vi "核查数据和日志信息出发送队列 (子VI).vi"() -> (0 "错误输出":errorcluster, 3 "核查数据上传":bool)   [LabVIEW 2016, in "数据传输系统.lvlib"]
uses:
  <vilib>/Utility/config.llb/NI_LVConfig.lvlib
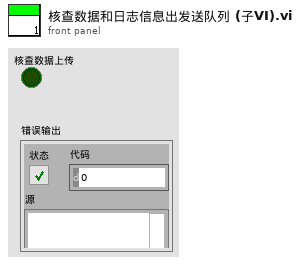
[diagram p1: front panel]
types:
  T1 = enum16{"质控数据", "操作日志", "仪器参数", "系统状态", "运行模式", "测量周期", "超标留样", "报警信息", "环境参数"}
  T2 = enum16{"空白测试", "跨度核查", "标样核查", "加标回收", "平行样", "集成干预"}
  T3 = typedef "NI_LVConfig.lvlib/Config Data RefNum.ctl" = refnum<k1>
  T4 = cluster{"PH":string[][], "CODCr":string[][], "氨氮":string[][], "CODMn":string[][], "总氮":string[][], "总磷":string[][], "电导率":string[][], "水温":string[][], "DO":string[][], "浊度":string[][], "叶绿素":string[][], "藻密度":string[][], "铜":string[][], "盐度":string[][], "水位":string[][], "流速":string[][], "瞬时流量":string[][], "累积流量":string[][]}
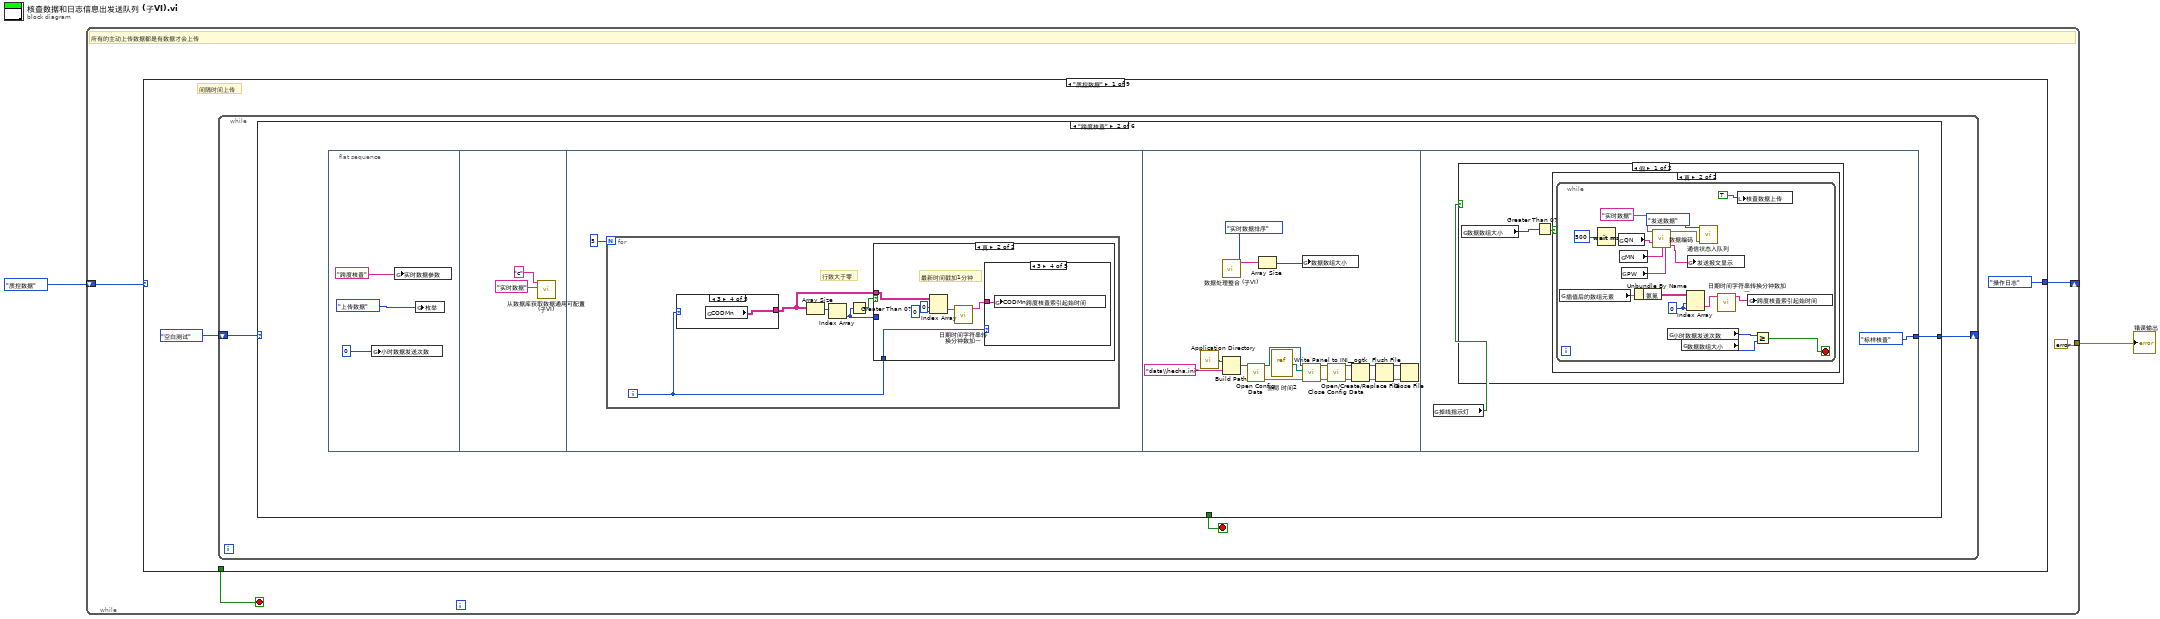
[diagram p0: block diagram]
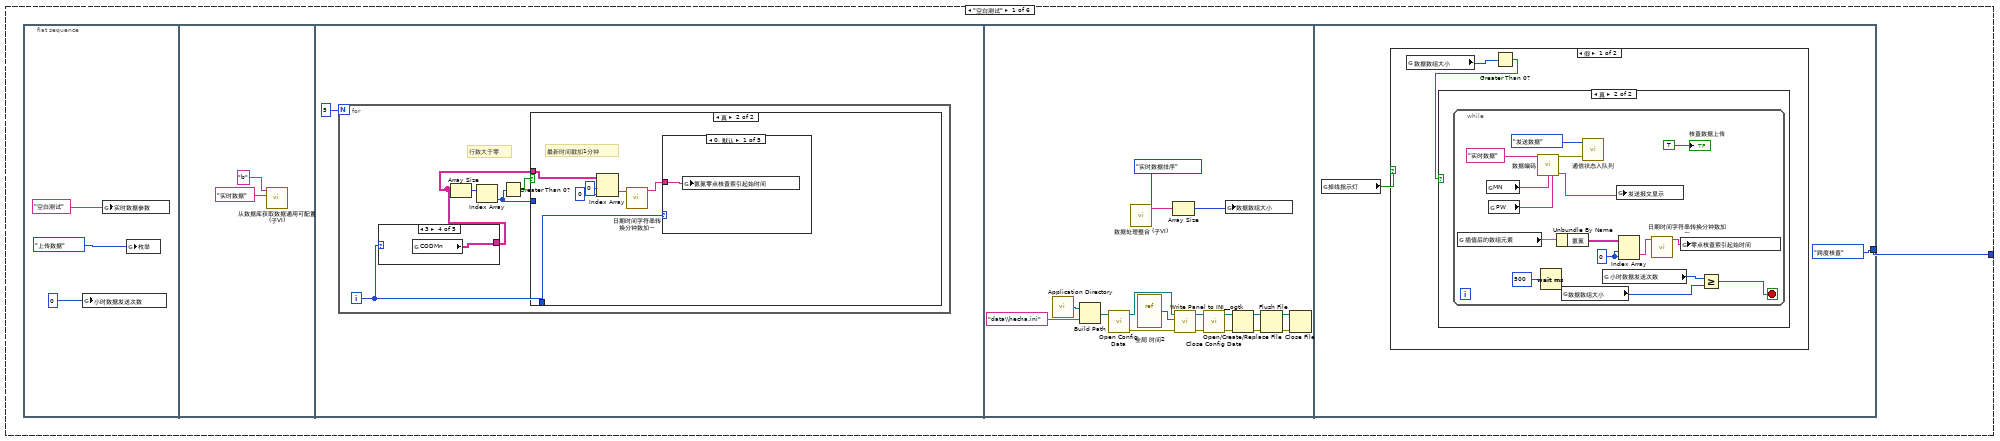
[diagram p2: hidden frame]
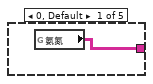
[diagram p3: hidden frame]
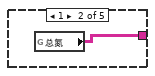
[diagram p4: hidden frame]
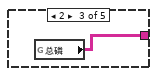
[diagram p5: hidden frame]
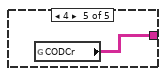
[diagram p6: hidden frame]
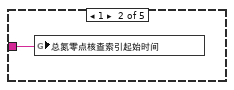
[diagram p8: hidden frame]
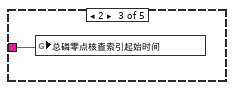
[diagram p9: hidden frame]
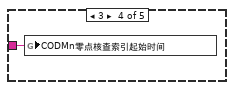
[diagram p10: hidden frame]
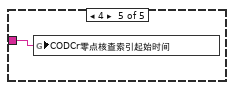
[diagram p11: hidden frame]
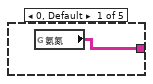
[diagram p14: hidden frame]
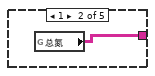
[diagram p15: hidden frame]
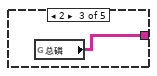
[diagram p16: hidden frame]
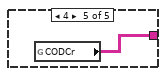
[diagram p17: hidden frame]
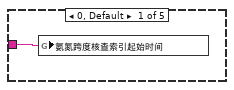
[diagram p19: hidden frame]
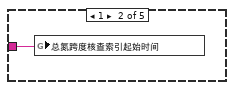
[diagram p20: hidden frame]
diagram:
  n1 = while "While循环" {
    shift-right: [w5] -> _
    shift-left: T1."质控数据" -> [w6]
    tunnel: [errorcluster {"status"=FALSE, "code"=0, "source"=""} ("错误输出")] -> w1
    stop <- w4 stop-if-true
    # "所有的主动上传数据都是有数据才会上传"
    n2 = case shown="\"质控数据\"" w6 {
      tunnel: [T1."操作日志" T1."仪器参数" T1."系统状态" T1."运行模式" T1."测量周期" T1."超标留样" T1."报警信息" T1."环境参数" T1."环境参数"] -> w5
      tunnel: [_ _ _ _ _ _ _ _ TRUE] -> w4
      frame "质控数据" {
        # "间隔时间上传"
        n3 = while {
          shift-right: [w9] -> _
          shift-left: T2."空白测试" -> [w10]
          stop <- w11 stop-if-true
          n4 = case shown="\"跨度核查\"" w10 {
            tunnel: [_ _ _ _ _ TRUE] -> w11
            tunnel: [w12 w77 w143 w173 w205 w266] -> w9
            frame "空白测试" {
              n5 = flat-sequence {
                tunnel: [T2."跨度核查"] -> w12
                frame #0 {
                  n6 = global write "全局 小时数据发送次数.vi" "小时数据发送次数"(0 ("小时数据发送次数")) -> ()
                  n7 = global write "全局 实时数据参数.vi" "实时数据参数"("空白测试") -> ()
                  n8 = global write "全局1.vi" "枚举"(enum16{"返回请求应答", "上传数据", "返回执行结果"}."上传数据" ("枚举")) -> ()
                }
                frame #1 {
                  n9 = call "从数据库获取数据通用可配置(子VI).vi"("table输入"="实时数据" ("新元素/子数组"), "列队名（唯一）"="b") -> ()  [unwired: 8 in, 2 out]
                }
                frame #2 {
                  n10 = for {
                    N: 5 -> [_]
                    i -> [w20]
                    # "行数大于零"
                    n11 = case shown="3" w20 {
                      tunnel: [w24 w25 w26 w27 w28] -> w19
                      frame 0, Default {
                        n12 = global read "全局 所有参数.vi" "氨氮"() -> (w24:string[][])
                      }
                      frame 1 {
                        n13 = global read "全局 所有参数.vi" "总氮"() -> (w25:string[][])
                      }
                      frame 2 {
                        n14 = global read "全局 所有参数.vi" "总磷"() -> (w26:string[][])
                      }
                      frame 3 {
                        n15 = global read "全局 所有参数.vi" "CODMn"() -> (w27:string[][])
                      }
                      frame 4 {
                        n16 = global read "全局 所有参数.vi" "CODCr"() -> (w28:string[][])
                      }
                    }
                    n17 = Array Size(array=w19) -> (size(s)=w22:i32[])
                    n18 = Index Array(array=w22) -> (element=w21:i32)  [unwired: 1 in]
                    n19 = Greater Than 0?(x=w21) -> (x > 0?=w23:bool)
                    n20 = case shown="真" w23 {
                      tunnel: w20 -> [_ w34]
                      tunnel: w21 -> [_ _]
                      tunnel: w19 -> [_ w32]
                      frame False {
                      }
                      frame True {
                        # "最新时间戳加1分钟"
                        n21 = Index Array(array=w32, index (row)=0 ("禁用的索引 (行)"), index (col)=0 ("禁用的索引 (列)")) -> (element=w31:string)
                        n22 = call "日期时间字符串转换分钟数加一.vi"("data[0]"=w31) -> ("日期/时间字符串"=w30:string)  [unwired: 10 in]
                        n23 = case shown="0, 默认" w34 {
                          tunnel: w30 -> [w35 w36 w37 w38 w39]
                          frame 0, Default {
                            n24 = global write "全局 时间2.vi" "氨氮零点核查索引起始时间"(w35) -> ()
                          }
                          frame 1 {
                            n25 = global write "全局 时间2.vi" "总氮零点核查索引起始时间"(w36) -> ()
                          }
                          frame 2 {
                            n26 = global write "全局 时间2.vi" "总磷零点核查索引起始时间"(w37) -> ()
                          }
                          frame 3 {
                            n27 = global write "全局 时间2.vi" "CODMn零点核查索引起始时间"(w38) -> ()
                          }
                          frame 4 {
                            n28 = global write "全局 时间2.vi" "CODCr零点核查索引起始时间"(w39) -> ()
                          }
                        }
                      }
                    }
                  }
                }
                frame #3 {
                  n29 = call <vilib>:"Application Directory.vi"() -> ("Application Directory"=w53:path)
                  n30 = Build Path(base path=w53, name or relative path="data\\hecha.ini" ("名称或相对路径")) -> (appended path=w51:path)
                  n31 = call <vilib>:"Open Config Data.vi"("configuration file path"=w51) -> ("error out"=w47:errorcluster, "refnum"=w50:T3)  [unwired: 8 in, 1 out]
                  n32 = call "数据处理整合 (子VI).vi"("枚举"=enum16{"实时数据排序", "小时数据排序"}."实时数据排序") -> ("已排序的数组"=w56:string[])  [unwired: 10 in]
                  n33 = vi-ref "全局 时间2.vi"() -> (w49:refnum<vi>)
                  n34 = Array Size(array=w56) -> (size(s)=w55:i32)
                  n35 = call <userlib>:"Write Panel to INI__ogtk.vi"("error in (no error)"=w47, "VI ref"=w49, "refnum"=w50) -> ("error out"=w46:errorcluster, "refnum out"=w48:T3)  [unwired: 7 in]
                  n36 = call <vilib>:"Close Config Data.vi"("error in (no error)"=w46, "refnum"=w48) -> ("error out"=w41:errorcluster, "file path"=w40:path)  [unwired: 8 in]
                  n37 = global write "全局 数据数组大小.vi" "数据数组大小"(w55) -> ()
                  n38 = Open/Create/Replace File(file path (use dialog)=w40, error in=w41) -> (refnum out=w44:refnum<file>, error out=w45:errorcluster)  [unwired: 4 in, 1 out]
                  n39 = Flush File(refnum=w44, error in=w45) -> (refnum out=w43:refnum<file>, error out=w42:errorcluster)
                  n40 = Close File(refnum=w43, error in=w42) -> ()  [unwired: 2 out]
                }
                frame #4 {
                  n41 = global read "全局 数据发送重叠.vi" "掉线指示灯"() -> (w58:bool)
                  n42 = case shown="假" w58 {
                    frame False {
                      n43 = global read "全局 数据数组大小.vi" "数据数组大小"() -> (w60:i32)
                      n44 = Greater Than 0?(x=w60) -> (x > 0?=w59:bool)
                      n45 = case shown="真" w59 {
                        frame False {
                        }
                        frame True {
                          n46 = while {
                            stop <- w62 stop-if-true
                            w71 = 0 ("禁用的索引 (列)")
                            n47 = global read "插值后的新数组.vi" "插值后的数组元素"() -> (w75:T4)
                            n48 = global read "断电保存全局.vi" "MN"() -> (w68:string)
                            n49 = global read "断电保存全局.vi" "PW"() -> (w67:string)
                            n50 = call "数据编码.vi"("table输入"="实时数据" ("新元素/子数组"), "MN"=w68, "PW"=w67) -> ("错误常量"=w66:errorcluster, "通讯包字符串"=w70:string)  [unwired: 11 in]
                            n51 = Wait (ms)(milliseconds to wait=u32 500 ("等待时间（毫秒）")) -> ()  [unwired: 1 out]
                            n52 = Unbundle By Name(w75) -> ("氨氮"=w74:string[][])
                            n53 = global read "全局 数据数组大小.vi" "数据数组大小"() -> (w65:i32)
                            n54 = call "通信状态入队列.vi"("错误输入（无错误）"=w66, "枚举"=enum16{"打开连接", "发送数据", "读取数据", "数据处理", "关闭连接"}."发送数据") -> ()  [unwired: 9 in, 1 out]
                            n55 = global read "全局 小时数据发送次数.vi" "小时数据发送次数"() -> (w63:i32)
                            n56 = global write "全局1.vi" "发送报文显示"(w70) -> ()
                            n57 = Index Array(array=w74, index (row)=w71, index (col)=w71) -> (element=w73:string)
                            n58 = call "日期时间字符串转换分钟数加一.vi"("data[0]"=w73) -> ("日期/时间字符串"=w72:string)  [unwired: 10 in]
                            n59 = global write "全局 时间2.vi" "零点核查索引起始时间"(w72) -> ()
                            n60 = Greater Or Equal?(x=w63, y=w65) -> (x >= y?=w62:bool)
                            "核查数据上传" <- TRUE ("数据上传")
                          }
                        }
                      }
                    }
                    frame True {
                    }
                  }
                }
              }
            }
            frame "跨度核查" {
              n61 = flat-sequence {
                tunnel: [T2."标样核查"] -> w77
                frame #0 {
                  n62 = global write "全局 小时数据发送次数.vi" "小时数据发送次数"(0 ("小时数据发送次数")) -> ()
                  n63 = global write "全局 实时数据参数.vi" "实时数据参数"("跨度核查") -> ()
                  n64 = global write "全局1.vi" "枚举"(enum16{"返回请求应答", "上传数据", "返回执行结果"}."上传数据" ("枚举")) -> ()
                }
                frame #1 {
                  n65 = call "从数据库获取数据通用可配置(子VI).vi"("table输入"="实时数据" ("新元素/子数组"), "列队名（唯一）"="c") -> ()  [unwired: 8 in, 2 out]
                }
                frame #2 {
                  n66 = for {
                    N: 5 -> [_]
                    i -> [w84]
                    # "行数大于零"
                    n67 = case shown="3" w84 {
                      tunnel: [w89 w90 w91 w92 w93] -> w85
                      frame 0, Default {
                        n68 = global read "全局 所有参数.vi" "氨氮"() -> (w89:string[][])
                      }
                      frame 1 {
                        n69 = global read "全局 所有参数.vi" "总氮"() -> (w90:string[][])
                      }
                      frame 2 {
                        n70 = global read "全局 所有参数.vi" "总磷"() -> (w91:string[][])
                      }
                      frame 3 {
                        n71 = global read "全局 所有参数.vi" "CODMn"() -> (w92:string[][])
                      }
                      frame 4 {
                        n72 = global read "全局 所有参数.vi" "CODCr"() -> (w93:string[][])
                      }
                    }
                    n73 = Array Size(array=w85) -> (size(s)=w87:i32[])
                    n74 = Index Array(array=w87) -> (element=w86:i32)  [unwired: 1 in]
                    n75 = Greater Than 0?(x=w86) -> (x > 0?=w88:bool)
                    n76 = case shown="真" w88 {
                      tunnel: w84 -> [_ w99]
                      tunnel: w86 -> [_ _]
                      tunnel: w85 -> [_ w97]
                      frame False {
                      }
                      frame True {
                        # "最新时间戳加1分钟"
                        n77 = Index Array(array=w97, index (row)=0 ("禁用的索引 (行)"), index (col)=0 ("禁用的索引 (列)")) -> (element=w96:string)
                        n78 = call "日期时间字符串转换分钟数加一.vi"("data[0]"=w96) -> ("日期/时间字符串"=w95:string)  [unwired: 10 in]
                        n79 = case shown="3" w99 {
                          tunnel: w95 -> [w100 w101 w102 w103 w104]
                          frame 0, Default {
                            n80 = global write "全局 时间2.vi" "氨氮跨度核查索引起始时间"(w100) -> ()
                          }
                          frame 1 {
                            n81 = global write "全局 时间2.vi" "总氮跨度核查索引起始时间"(w101) -> ()
                          }
                          frame 2 {
                            n82 = global write "全局 时间2.vi" "总磷跨度核查索引起始时间"(w102) -> ()
                          }
                          frame 3 {
                            n83 = global write "全局 时间2.vi" "CODMn跨度核查索引起始时间"(w103) -> ()
                          }
                          frame 4 {
                            n84 = global write "全局 时间2.vi" "CODCr跨度核查索引起始时间"(w104) -> ()
                          }
                        }
                      }
                    }
                  }
                }
                frame #3 {
                  n85 = call <vilib>:"Application Directory.vi"() -> ("Application Directory"=w118:path)
                  n86 = call "数据处理整合 (子VI).vi"("枚举"=enum16{"实时数据排序", "小时数据排序"}."实时数据排序") -> ("已排序的数组"=w121:string[])  [unwired: 10 in]
                  n87 = Build Path(base path=w118, name or relative path="data\\hecha.ini" ("名称或相对路径")) -> (appended path=w116:path)
                  n88 = call <vilib>:"Open Config Data.vi"("configuration file path"=w116) -> ("error out"=w112:errorcluster, "refnum"=w115:T3)  [unwired: 8 in, 1 out]
                  n89 = Array Size(array=w121) -> (size(s)=w120:i32)
                  n90 = vi-ref "全局 时间2.vi"() -> (w114:refnum<vi>)
                  n91 = global write "全局 数据数组大小.vi" "数据数组大小"(w120) -> ()
                  n92 = call <userlib>:"Write Panel to INI__ogtk.vi"("error in (no error)"=w112, "VI ref"=w114, "refnum"=w115) -> ("error out"=w111:errorcluster, "refnum out"=w113:T3)  [unwired: 7 in]
                  n93 = call <vilib>:"Close Config Data.vi"("error in (no error)"=w111, "refnum"=w113) -> ("error out"=w106:errorcluster, "file path"=w105:path)  [unwired: 8 in]
                  n94 = Open/Create/Replace File(file path (use dialog)=w105, error in=w106) -> (refnum out=w109:refnum<file>, error out=w110:errorcluster)  [unwired: 4 in, 1 out]
                  n95 = Flush File(refnum=w109, error in=w110) -> (refnum out=w108:refnum<file>, error out=w107:errorcluster)
                  n96 = Close File(refnum=w108, error in=w107) -> ()  [unwired: 2 out]
                }
                frame #4 {
                  n97 = global read "全局 数据发送重叠.vi" "掉线指示灯"() -> (w123:bool)
                  n98 = case shown="假" w123 {
                    frame False {
                      n99 = global read "全局 数据数组大小.vi" "数据数组大小"() -> (w125:i32)
                      n100 = Greater Than 0?(x=w125) -> (x > 0?=w124:bool)
                      n101 = case shown="真" w124 {
                        frame False {
                        }
                        frame True {
                          n102 = while {
                            stop <- w126 stop-if-true
                            w137 = 0 ("禁用的索引 (列)")
                            n103 = global read "插值后的新数组.vi" "插值后的数组元素"() -> (w141:T4)
                            n104 = Wait (ms)(milliseconds to wait=u32 500 ("等待时间（毫秒）")) -> ()  [unwired: 1 out]
                            n105 = global read "全局1.vi" "QN"() -> (w136:string)
                            n106 = global read "断电保存全局.vi" "MN"() -> (w133:string)
                            n107 = global read "断电保存全局.vi" "PW"() -> (w132:string)
                            n108 = Unbundle By Name(w141) -> ("氨氮"=w140:string[][])
                            n109 = call "数据编码.vi"("table输入"="实时数据" ("新元素/子数组"), "QN"=w136, "MN"=w133, "PW"=w132) -> ("错误常量"=w130:errorcluster, "通讯包字符串"=w131:string)  [unwired: 10 in]
                            n110 = global read "全局 小时数据发送次数.vi" "小时数据发送次数"() -> (w127:i32)
                            n111 = global read "全局 数据数组大小.vi" "数据数组大小"() -> (w128:i32)
                            n112 = Index Array(array=w140, index (row)=w137, index (col)=w137) -> (element=w139:string)
                            n113 = global write "全局1.vi" "发送报文显示"(w131) -> ()
                            n114 = call "通信状态入队列.vi"("错误输入（无错误）"=w130, "枚举"=enum16{"打开连接", "发送数据", "读取数据", "数据处理", "关闭连接"}."发送数据") -> ()  [unwired: 9 in, 1 out]
                            n115 = call "日期时间字符串转换分钟数加一.vi"("data[0]"=w139) -> ("日期/时间字符串"=w138:string)  [unwired: 10 in]
                            n116 = local write "核查数据上传"(TRUE ("数据上传")) -> ()
                            n117 = global write "全局 时间2.vi" "跨度核查索引起始时间"(w138) -> ()
                            n118 = Greater Or Equal?(x=w127, y=w128) -> (x >= y?=w126:bool)
                          }
                        }
                      }
                    }
                    frame True {
                    }
                  }
                }
              }
            }
            frame "标样核查" {
              n119 = flat-sequence {
                tunnel: [T2."加标回收"] -> w143
                frame #0 {
                  n120 = global write "全局 小时数据发送次数.vi" "小时数据发送次数"(0 ("小时数据发送次数")) -> ()
                  n121 = global write "全局 实时数据参数.vi" "实时数据参数"("核查数据") -> ()
                  n122 = global write "全局1.vi" "枚举"(enum16{"返回请求应答", "上传数据", "返回执行结果"}."上传数据" ("枚举")) -> ()
                }
                frame #1 {
                  n123 = call "从数据库获取数据通用可配置(子VI).vi"("table输入"="实时数据" ("新元素/子数组"), "列队名（唯一）"="n") -> ()  [unwired: 8 in, 2 out]
                }
                frame #2 {
                  n124 = call "数据处理整合 (子VI).vi"("枚举"=enum16{"实时数据排序", "小时数据排序"}."实时数据排序") -> ("已排序的数组"=w151:string[])  [unwired: 10 in]
                  n125 = Array Size(array=w151) -> (size(s)=w150:i32)
                  n126 = global write "全局 数据数组大小.vi" "数据数组大小"(w150) -> ()
                }
                frame #3 {
                  n127 = global read "全局 数据发送重叠.vi" "掉线指示灯"() -> (w153:bool)
                  n128 = case shown="假" w153 {
                    frame False {
                      n129 = global read "全局 数据数组大小.vi" "数据数组大小"() -> (w155:i32)
                      n130 = Greater Than 0?(x=w155) -> (x > 0?=w154:bool)
                      n131 = case shown="真" w154 {
                        frame False {
                        }
                        frame True {
                          n132 = while {
                            stop <- w157 stop-if-true
                            w167 = 0 ("禁用的索引 (列)")
                            n133 = global read "插值后的新数组.vi" "插值后的数组元素"() -> (w171:T4)
                            n134 = global read "全局1.vi" "QN"() -> (w166:string)
                            n135 = global read "断电保存全局.vi" "MN"() -> (w162:string)
                            n136 = global read "断电保存全局.vi" "PW"() -> (w161:string)
                            n137 = Unbundle By Name(w171) -> ("氨氮"=w170:string[][])
                            n138 = call "数据编码.vi"("table输入"="实时数据" ("新元素/子数组"), "QN"=w166, "MN"=w162, "PW"=w161) -> ("错误常量"=w160:errorcluster, "通讯包字符串"=w165:string)  [unwired: 10 in]
                            n139 = global read "全局 小时数据发送次数.vi" "小时数据发送次数"() -> (w158:i32)
                            n140 = global write "全局1.vi" "发送报文显示"(w165) -> ()
                            n141 = global read "全局 数据数组大小.vi" "数据数组大小"() -> (w159:i32)
                            n142 = Index Array(array=w170, index (row)=w167, index (col)=w167) -> (element=w169:string)
                            n143 = call "通信状态入队列.vi"("错误输入（无错误）"=w160, "枚举"=enum16{"打开连接", "发送数据", "读取数据", "数据处理", "关闭连接"}."发送数据") -> ()  [unwired: 9 in, 1 out]
                            n144 = call "日期时间字符串转换分钟数加一.vi"("data[0]"=w169) -> ("日期/时间字符串"=w168:string)  [unwired: 10 in]
                            n145 = local write "核查数据上传"(TRUE ("数据上传")) -> ()
                            n146 = global write "全局 时间2.vi" "标样核查索引起始时间"(w168) -> ()
                            n147 = Greater Or Equal?(x=w158, y=w159) -> (x >= y?=w157:bool)
                            n148 = Wait (ms)(milliseconds to wait=u32 500 ("等待时间（毫秒）")) -> ()  [unwired: 1 out]
                          }
                        }
                      }
                    }
                    frame True {
                    }
                  }
                }
              }
            }
            frame "加标回收" {
              n149 = flat-sequence {
                tunnel: [T2."平行样"] -> w173
                frame #0 {
                  n150 = global write "全局 小时数据发送次数.vi" "小时数据发送次数"(0 ("小时数据发送次数")) -> ()
                  n151 = global write "全局 实时数据参数.vi" "实时数据参数"("加标回收测试") -> ()
                  n152 = global write "全局1.vi" "枚举"(enum16{"返回请求应答", "上传数据", "返回执行结果"}."上传数据" ("枚举")) -> ()
                }
                frame #1 {
                  n153 = call "从数据库获取数据通用可配置(子VI).vi"("table输入"="加标回收" ("新元素/子数组"), "列队名（唯一）"="d") -> ()  [unwired: 8 in, 2 out]
                }
                frame #2 {
                  n154 = call "加标回收数据处理整合 (子VI).vi"("枚举"=enum16{"实时数据排序", "小时数据排序"}."实时数据排序") -> ("已排序的数组"=w180:string[])  [unwired: 10 in]
                  n155 = Array Size(array=w180) -> (size(s)=w181:i32)
                  n156 = global write "全局 数据数组大小.vi" "数据数组大小"(w181) -> ()
                }
                frame #3 {
                  n157 = global read "全局 数据发送重叠.vi" "掉线指示灯"() -> (w183:bool)
                  n158 = case shown="假" w183 {
                    frame False {
                      n159 = global read "全局 数据数组大小.vi" "数据数组大小"() -> (w185:i32)
                      n160 = Greater Than 0?(x=w185) -> (x > 0?=w184:bool)
                      n161 = case shown="真" w184 {
                        frame False {
                        }
                        frame True {
                          n162 = while {
                            stop <- w187 stop-if-true
                            n163 = global read "全局 数据数组大小.vi" "数据数组大小"() -> (w200:i32)
                            n164 = global read "插值后的新数组.vi" "插值后的数组元素"() -> (w203:T4)
                            n165 = global read "全局1.vi" "QN"() -> (w196:string)
                            n166 = global read "断电保存全局.vi" "MN"() -> (w192:string)
                            n167 = global read "断电保存全局.vi" "PW"() -> (w191:string)
                            n168 = Decrement(x=w200) -> (x-1=w199:i32)
                            n169 = call "数据编码.vi"("table输入"="实时数据" ("新元素/子数组"), "QN"=w196, "MN"=w192, "PW"=w191) -> ("错误常量"=w190:errorcluster, "通讯包字符串"=w195:string)  [unwired: 10 in]
                            n170 = Unbundle By Name(w203) -> ("氨氮"=w202:string[][])
                            n171 = global write "全局1.vi" "发送报文显示"(w195) -> ()
                            n172 = call "通信状态入队列.vi"("错误输入（无错误）"=w190, "枚举"=enum16{"打开连接", "发送数据", "读取数据", "数据处理", "关闭连接"}."发送数据") -> ()  [unwired: 9 in, 1 out]
                            n173 = global read "全局 小时数据发送次数.vi" "小时数据发送次数"() -> (w188:i32)
                            n174 = Index Array(array=w202, index (row)=w199, index (col)=0 ("禁用的索引 (列)")) -> (element=w198:string)
                            n175 = global read "全局 数据数组大小.vi" "数据数组大小"() -> (w189:i32)
                            n176 = call "日期时间字符串转换分钟数加一.vi"("data[0]"=w198) -> ("日期/时间字符串"=w197:string)  [unwired: 10 in]
                            n177 = local write "核查数据上传"(TRUE ("数据上传")) -> ()
                            n178 = global write "全局 时间2.vi" "加标回收索引起始时间"(w197) -> ()
                            n179 = Greater Or Equal?(x=w188, y=w189) -> (x >= y?=w187:bool)
                            n180 = Wait (ms)(milliseconds to wait=u32 500 ("等待时间（毫秒）")) -> ()  [unwired: 1 out]
                          }
                        }
                      }
                    }
                    frame True {
                    }
                  }
                }
              }
            }
            frame "平行样" {
              n181 = flat-sequence {
                tunnel: [T2."集成干预"] -> w205
                frame #0 {
                  n182 = global write "全局 小时数据发送次数.vi" "小时数据发送次数"(0 ("小时数据发送次数")) -> ()
                  n183 = global write "全局 实时数据参数.vi" "实时数据参数"("平行样测试") -> ()
                  n184 = global write "全局1.vi" "枚举"(enum16{"返回请求应答", "上传数据", "返回执行结果"}."上传数据" ("枚举")) -> ()
                }
                frame #1 {
                  n185 = call "从数据库获取数据通用可配置(子VI).vi"("table输入"="平行样测试" ("新元素/子数组"), "列队名（唯一）"="e") -> ()  [unwired: 8 in, 2 out]
                }
                frame #2 {
                  n186 = for {
                    N: 5 -> [_]
                    i -> [w212]
                    # "行数大于零"
                    n187 = case shown="3" w212 {
                      tunnel: [w217 w218 w219 w220 w221] -> w213
                      frame 0, Default {
                        n188 = global read "全局 所有参数.vi" "氨氮"() -> (w217:string[][])
                      }
                      frame 1 {
                        n189 = global read "全局 所有参数.vi" "总氮"() -> (w218:string[][])
                      }
                      frame 2 {
                        n190 = global read "全局 所有参数.vi" "总磷"() -> (w219:string[][])
                      }
                      frame 3 {
                        n191 = global read "全局 所有参数.vi" "CODMn"() -> (w220:string[][])
                      }
                      frame 4 {
                        n192 = global read "全局 所有参数.vi" "CODCr"() -> (w221:string[][])
                      }
                    }
                    n193 = Array Size(array=w213) -> (size(s)=w215:i32[])
                    n194 = Index Array(array=w215) -> (element=w214:i32)  [unwired: 1 in]
                    n195 = Greater Than 0?(x=w214) -> (x > 0?=w216:bool)
                    n196 = case shown="真" w216 {
                      tunnel: w212 -> [_ w227]
                      tunnel: w214 -> [_ _]
                      tunnel: w213 -> [_ w225]
                      frame False {
                      }
                      frame True {
                        # "最新时间戳加1分钟"
                        n197 = Index Array(array=w225, index (row)=0 ("禁用的索引 (行)"), index (col)=0 ("禁用的索引 (列)")) -> (element=w224:string)
                        n198 = call "日期时间字符串转换分钟数加一.vi"("data[0]"=w224) -> ("日期/时间字符串"=w223:string)  [unwired: 10 in]
                        n199 = case shown="0, 默认" w227 {
                          tunnel: w223 -> [w228 w229 w230 w231 w232]
                          frame 0, Default {
                            n200 = global write "全局 时间2.vi" "氨氮平行样索引起始时间"(w228) -> ()
                          }
                          frame 1 {
                            n201 = global write "全局 时间2.vi" "总氮平行样索引起始时间"(w229) -> ()
                          }
                          frame 2 {
                            n202 = global write "全局 时间2.vi" "总磷平行样索引起始时间"(w230) -> ()
                          }
                          frame 3 {
                            n203 = global write "全局 时间2.vi" "CODMn平行样索引起始时间"(w231) -> ()
                          }
                          frame 4 {
                            n204 = global write "全局 时间2.vi" "CODCr平行样索引起始时间"(w232) -> ()
                          }
                        }
                      }
                    }
                  }
                }
                frame #3 {
                  n205 = call "数据处理整合 (子VI).vi"("枚举"=enum16{"实时数据排序", "小时数据排序"}."实时数据排序") -> ("已排序的数组"=w249:string[])  [unwired: 10 in]
                  n206 = Array Size(array=w249) -> (size(s)=w248:i32)
                  n207 = call <vilib>:"Application Directory.vi"() -> ("Application Directory"=w246:path)
                  n208 = Build Path(base path=w246, name or relative path="data\\hecha.ini" ("名称或相对路径")) -> (appended path=w244:path)
                  n209 = global write "全局 数据数组大小.vi" "数据数组大小"(w248) -> ()
                  n210 = call <vilib>:"Open Config Data.vi"("configuration file path"=w244) -> ("error out"=w240:errorcluster, "refnum"=w243:T3)  [unwired: 8 in, 1 out]
                  n211 = vi-ref "全局 时间2.vi"() -> (w242:refnum<vi>)
                  n212 = call <userlib>:"Write Panel to INI__ogtk.vi"("error in (no error)"=w240, "VI ref"=w242, "refnum"=w243) -> ("error out"=w239:errorcluster, "refnum out"=w241:T3)  [unwired: 7 in]
                  n213 = call <vilib>:"Close Config Data.vi"("error in (no error)"=w239, "refnum"=w241) -> ("error out"=w234:errorcluster, "file path"=w233:path)  [unwired: 8 in]
                  n214 = Open/Create/Replace File(file path (use dialog)=w233, error in=w234) -> (refnum out=w237:refnum<file>, error out=w238:errorcluster)  [unwired: 4 in, 1 out]
                  n215 = Flush File(refnum=w237, error in=w238) -> (refnum out=w236:refnum<file>, error out=w235:errorcluster)
                  n216 = Close File(refnum=w236, error in=w235) -> ()  [unwired: 2 out]
                }
                frame #4 {
                  n217 = global read "全局 数据发送重叠.vi" "掉线指示灯"() -> (w250:bool)
                  n218 = case shown="假" w250 {
                    frame False {
                      n219 = global read "全局 数据数组大小.vi" "数据数组大小"() -> (w253:i32)
                      n220 = Greater Than 0?(x=w253) -> (x > 0?=w252:bool)
                      n221 = case shown="真" w252 {
                        frame False {
                        }
                        frame True {
                          n222 = while {
                            stop <- w255 stop-if-true
                            n223 = global read "全局1.vi" "QN"() -> (w264:string)
                            n224 = global read "断电保存全局.vi" "MN"() -> (w260:string)
                            n225 = global read "断电保存全局.vi" "PW"() -> (w259:string)
                            n226 = global read "全局 小时数据发送次数.vi" "小时数据发送次数"() -> (w256:i32)
                            n227 = global read "全局 数据数组大小.vi" "数据数组大小"() -> (w257:i32)
                            n228 = call "数据编码.vi"("table输入"="实时数据" ("新元素/子数组"), "QN"=w264, "MN"=w260, "PW"=w259) -> ("错误常量"=w258:errorcluster, "通讯包字符串"=w263:string)  [unwired: 10 in]
                            n229 = local write "核查数据上传"(TRUE ("数据上传")) -> ()
                            n230 = global write "全局1.vi" "发送报文显示"(w263) -> ()
                            n231 = call "通信状态入队列.vi"("错误输入（无错误）"=w258, "枚举"=enum16{"打开连接", "发送数据", "读取数据", "数据处理", "关闭连接"}."发送数据") -> ()  [unwired: 9 in, 1 out]
                            n232 = Greater Or Equal?(x=w256, y=w257) -> (x >= y?=w255:bool)
                            n233 = Wait (ms)(milliseconds to wait=u32 500 ("等待时间（毫秒）")) -> ()  [unwired: 1 out]
                          }
                        }
                      }
                    }
                    frame True {
                    }
                  }
                }
              }
            }
            frame "集成干预" {
              n234 = flat-sequence {
                tunnel: [T2."集成干预"] -> w266
                frame #0 {
                  n235 = global write "全局 小时数据发送次数.vi" "小时数据发送次数"(0 ("小时数据发送次数")) -> ()
                  n236 = global write "全局 实时数据参数.vi" "实时数据参数"("集成干预测试") -> ()
                  n237 = global write "全局1.vi" "枚举"(enum16{"返回请求应答", "上传数据", "返回执行结果"}."上传数据" ("枚举")) -> ()
                }
                frame #1 {
                  n238 = call "从数据库获取数据通用可配置(子VI).vi"("table输入"="集成干预测试" ("新元素/子数组"), "列队名（唯一）"="f") -> ()  [unwired: 8 in, 2 out]
                }
                frame #2 {
                  n239 = for {
                    N: 10 -> [_]
                    i -> [w274]
                    # "行数大于零"
                    n240 = case shown="9" w274 {
                      tunnel: [w279 w280 w281 w282 w283 w284 w285 w286 w287 w288] -> w275
                      frame 0, Default {
                        n241 = global read "全局 所有参数.vi" "氨氮"() -> (w279:string[][])
                      }
                      frame 1 {
                        n242 = global read "全局 所有参数.vi" "总氮"() -> (w280:string[][])
                      }
                      frame 2 {
                        n243 = global read "全局 所有参数.vi" "总磷"() -> (w281:string[][])
                      }
                      frame 3 {
                        n244 = global read "全局 所有参数.vi" "CODMn"() -> (w282:string[][])
                      }
                      frame 4 {
                        n245 = global read "全局 所有参数.vi" "CODCr"() -> (w283:string[][])
                      }
                      frame 5 {
                        n246 = global read "全局 所有参数.vi" "DO"() -> (w284:string[][])
                      }
                      frame 6 {
                        n247 = global read "全局 所有参数.vi" "PH"() -> (w285:string[][])
                      }
                      frame 7 {
                        n248 = global read "全局 所有参数.vi" "电导率"() -> (w286:string[][])
                      }
                      frame 8 {
                        n249 = global read "全局 所有参数.vi" "水温"() -> (w287:string[][])
                      }
                      frame 9 {
                        n250 = global read "全局 所有参数.vi" "浊度"() -> (w288:string[][])
                      }
                    }
                    n251 = Array Size(array=w275) -> (size(s)=w277:i32[])
                    n252 = Index Array(array=w277) -> (element=w276:i32)  [unwired: 1 in]
                    n253 = Greater Than 0?(x=w276) -> (x > 0?=w278:bool)
                    n254 = case shown="真" w278 {
                      tunnel: w274 -> [_ w294]
                      tunnel: w276 -> [_ _]
                      tunnel: w275 -> [_ w292]
                      frame False {
                      }
                      frame True {
                        # "最新时间戳加1分钟"
                        n255 = Index Array(array=w292, index (row)=0 ("禁用的索引 (行)"), index (col)=0 ("禁用的索引 (列)")) -> (element=w291:string)
                        n256 = call "日期时间字符串转换分钟数加一.vi"("data[0]"=w291) -> ("日期/时间字符串"=w290:string)  [unwired: 10 in]
                        n257 = case shown="9" w294 {
                          tunnel: w290 -> [w295 w296 w297 w298 w299 w300 w301 w302 w303 w304]
                          frame 0, Default {
                            n258 = global write "全局 时间2.vi" "氨氮集成干预索引起始时间"(w295) -> ()
                          }
                          frame 1 {
                            n259 = global write "全局 时间2.vi" "总氮集成干预索引起始时间"(w296) -> ()
                          }
                          frame 2 {
                            n260 = global write "全局 时间2.vi" "总磷集成干预索引起始时间"(w297) -> ()
                          }
                          frame 3 {
                            n261 = global write "全局 时间2.vi" "CODMn集成干预索引起始时间"(w298) -> ()
                          }
                          frame 4 {
                            n262 = global write "全局 时间2.vi" "CODCr集成干预索引起始时间"(w299) -> ()
                          }
                          frame 5 {
                            n263 = global write "全局 时间2.vi" "DO集成干预索引起始时间"(w300) -> ()
                          }
                          frame 6 {
                            n264 = global write "全局 时间2.vi" "PH集成干预索引起始时间"(w301) -> ()
                          }
                          frame 7 {
                            n265 = global write "全局 时间2.vi" "比电导率集成干预索引起始时间"(w302) -> ()
                          }
                          frame 8 {
                            n266 = global write "全局 时间2.vi" "水温集成干预索引起始时间"(w303) -> ()
                          }
                          frame 9 {
                            n267 = global write "全局 时间2.vi" "浊度集成干预索引起始时间"(w304) -> ()
                          }
                        }
                      }
                    }
                  }
                }
                frame #3 {
                  n268 = call "数据处理整合 (子VI).vi"("枚举"=enum16{"实时数据排序", "小时数据排序"}."实时数据排序") -> ("已排序的数组"=w321:string[])  [unwired: 10 in]
                  n269 = Array Size(array=w321) -> (size(s)=w320:i32)
                  n270 = call <vilib>:"Application Directory.vi"() -> ("Application Directory"=w318:path)
                  n271 = Build Path(base path=w318, name or relative path="data\\hecha.ini" ("名称或相对路径")) -> (appended path=w316:path)
                  n272 = global write "全局 数据数组大小.vi" "数据数组大小"(w320) -> ()
                  n273 = call <vilib>:"Open Config Data.vi"("configuration file path"=w316) -> ("error out"=w312:errorcluster, "refnum"=w315:T3)  [unwired: 8 in, 1 out]
                  n274 = vi-ref "全局 时间2.vi"() -> (w314:refnum<vi>)
                  n275 = call <userlib>:"Write Panel to INI__ogtk.vi"("error in (no error)"=w312, "VI ref"=w314, "refnum"=w315) -> ("error out"=w311:errorcluster, "refnum out"=w313:T3)  [unwired: 7 in]
                  n276 = call <vilib>:"Close Config Data.vi"("error in (no error)"=w311, "refnum"=w313) -> ("error out"=w306:errorcluster, "file path"=w305:path)  [unwired: 8 in]
                  n277 = Open/Create/Replace File(file path (use dialog)=w305, error in=w306) -> (refnum out=w309:refnum<file>, error out=w310:errorcluster)  [unwired: 4 in, 1 out]
                  n278 = Flush File(refnum=w309, error in=w310) -> (refnum out=w308:refnum<file>, error out=w307:errorcluster)
                  n279 = Close File(refnum=w308, error in=w307) -> ()  [unwired: 2 out]
                }
                frame #4 {
                  n280 = global read "全局 数据发送重叠.vi" "掉线指示灯"() -> (w323:bool)
                  n281 = case shown="假" w323 {
                    frame False {
                      n282 = global read "全局 数据数组大小.vi" "数据数组大小"() -> (w325:i32)
                      n283 = Greater Than 0?(x=w325) -> (x > 0?=w324:bool)
                      n284 = case shown="真" w324 {
                        frame False {
                        }
                        frame True {
                          n285 = while {
                            stop <- w327 stop-if-true
                            n286 = global read "全局1.vi" "QN"() -> (w336:string)
                            n287 = global read "断电保存全局.vi" "MN"() -> (w331:string)
                            n288 = global read "断电保存全局.vi" "PW"() -> (w330:string)
                            n289 = global read "全局 数据数组大小.vi" "数据数组大小"() -> (w329:i32)
                            n290 = global read "全局 小时数据发送次数.vi" "小时数据发送次数"() -> (w328:i32)
                            n291 = call "数据编码.vi"("table输入"="实时数据" ("新元素/子数组"), "QN"=w336, "MN"=w331, "PW"=w330) -> ("错误常量"=w332:errorcluster, "通讯包字符串"=w335:string)  [unwired: 10 in]
                            n292 = local write "核查数据上传"(TRUE ("数据上传")) -> ()
                            n293 = call "通信状态入队列.vi"("错误输入（无错误）"=w332, "枚举"=enum16{"打开连接", "发送数据", "读取数据", "数据处理", "关闭连接"}."发送数据") -> ()  [unwired: 9 in, 1 out]
                            n294 = global write "全局1.vi" "发送报文显示"(w335) -> ()
                            n295 = Greater Or Equal?(x=w328, y=w329) -> (x >= y?=w327:bool)
                            n296 = Wait (ms)(milliseconds to wait=u32 500 ("等待时间（毫秒）")) -> ()  [unwired: 1 out]
                          }
                        }
                      }
                    }
                    frame True {
                    }
                  }
                }
              }
            }
          }
        }
      }
      frame "操作日志" {
        # "间隔时间上传"
        # "直接1分钟查询 一次,有数据就按数据上传,没数据就不上传,在数据发送那边有做处理"
        n297 = flat-sequence {
          frame #0 {
            # "时间"
            n298 = global write "全局 小时数据发送次数.vi" "小时数据发送次数"(0 ("小时数据发送次数")) -> ()
            n299 = call "日志信息主动发送(子VI).vi"() -> ()  [unwired: 12 in]
            n300 = global write "全局1.vi" "枚举"(enum16{"返回请求应答", "上传数据", "返回执行结果"}."上传数据" ("枚举")) -> ()
          }
          frame #1 {
            n301 = call "获取操作日志 (子VI).vi"("table输入"="操作日志") -> ()  [unwired: 11 in]
          }
          frame #2 {
            n302 = call "数据处理整合 (子VI).vi"("枚举"=enum16{"实时数据排序", "小时数据排序"}."实时数据排序") -> ("已排序的数组"=w344:string[])  [unwired: 10 in]
            n303 = Array Size(array=w344) -> (size(s)=w343:i32)
            n304 = global write "全局 数据数组大小.vi" "数据数组大小"(w343) -> ()
          }
          frame #3 {
            # "判定是否存表"
            n305 = global read "全局 数据发送重叠.vi" "掉线指示灯"() -> (w345:bool)
            n306 = case shown="假" w345 {
              frame False {
                n307 = global read "全局 数据数组大小.vi" "数据数组大小"() -> (w346:i32)
                n308 = Greater Than 0?(x=w346) -> (x > 0?=w347:bool)
                n309 = case shown="真" w347 {
                  frame False {
                  }
                  frame True {
                    n310 = while {
                      stop <- w349 stop-if-true
                      n311 = global read "全局 小时数据发送次数.vi" "小时数据发送次数"() -> (w360:i32)
                      n312 = local write "核查数据上传"(TRUE ("数据上传")) -> ()
                      n313 = Get Date/Time In Seconds() -> (seconds since 1Jan1904=w364:timestamp)
                      n314 = Increment(x=w360) -> (x+1=w359:i32)
                      n315 = Format Date/Time String(time format string (%c)="%Y%m%d%H%M%S%3u" ("时间格式字符串(%c)"), seconds (now)=w364) -> (date/time string=w363:string)  [unwired: 1 in]
                      n316 = global write "全局 小时数据发送次数.vi" "小时数据发送次数"(w359) -> ()
                      n317 = Search and Replace String(input string=w363, search string="." ("搜索字符串")) -> (result string=w361:string)  [unwired: 6 in, 3 out]
                      n318 = global read "断电保存全局.vi" "MN"() -> (w355:string)
                      n319 = global read "断电保存全局.vi" "PW"() -> (w354:string)
                      n320 = call "数据编码.vi"("table输入"="操作日志" ("新元素/子数组"), "QN"=w361, "MN"=w355, "PW"=w354) -> ("错误常量"=w353:errorcluster, "通讯包字符串"=w358:string)  [unwired: 10 in]
                      n321 = global read "全局 小时数据发送次数.vi" "小时数据发送次数"() -> (w350:i32)
                      n322 = global read "全局 数据数组大小.vi" "数据数组大小"() -> (w351:i32)
                      n323 = call "通信状态入队列.vi"("错误输入（无错误）"=w353, "枚举"=enum16{"打开连接", "发送数据", "读取数据", "数据处理", "关闭连接"}."发送数据") -> ()  [unwired: 9 in, 1 out]
                      n324 = global write "全局1.vi" "发送报文显示"(w358) -> ()
                      n325 = Decrement(x=w351) -> (x-1=w352:i32)
                      n326 = Greater Or Equal?(x=w350, y=w352) -> (x >= y?=w349:bool)
                      n327 = Wait (ms)(milliseconds to wait=u32 500 ("等待时间（毫秒）")) -> ()  [unwired: 1 out]
                    }
                  }
                }
              }
              frame True {
              }
            }
          }
        }
      }
      frame "仪器参数" {
        # "间隔时间上传"
        # "直接1分钟查询 一次,有数据就按数据上传,没数据就不上传,在数据发送那边有做处理"
        n328 = flat-sequence {
          frame #0 {
            # "时间"
            n329 = global write "全局 小时数据发送次数.vi" "小时数据发送次数"(0 ("小时数据发送次数")) -> ()
            n330 = call "日志信息主动发送(子VI).vi"() -> ()  [unwired: 12 in]
            n331 = global write "全局1.vi" "枚举"(enum16{"返回请求应答", "上传数据", "返回执行结果"}."上传数据" ("枚举")) -> ()
          }
          frame #1 {
            n332 = call "获取操作日志 (子VI).vi"("table输入"="仪器参数") -> ()  [unwired: 11 in]
          }
          frame #2 {
            n333 = call "数据处理整合 (子VI).vi"("枚举"=enum16{"实时数据排序", "小时数据排序"}."实时数据排序") -> ("已排序的数组"=w373:string[])  [unwired: 10 in]
            n334 = Array Size(array=w373) -> (size(s)=w372:i32)
            n335 = global write "全局 数据数组大小.vi" "数据数组大小"(w372) -> ()
          }
          frame #3 {
            # "判定是否存表"
            n336 = global read "全局 数据发送重叠.vi" "掉线指示灯"() -> (w374:bool)
            n337 = case shown="假" w374 {
              frame False {
                n338 = global read "全局 数据数组大小.vi" "数据数组大小"() -> (w375:i32)
                n339 = Greater Than 0?(x=w375) -> (x > 0?=w376:bool)
                n340 = case shown="真" w376 {
                  frame False {
                  }
                  frame True {
                    n341 = while {
                      stop <- w377 stop-if-true
                      n342 = global read "全局 小时数据发送次数.vi" "小时数据发送次数"() -> (w389:i32)
                      n343 = local write "核查数据上传"(TRUE ("数据上传")) -> ()
                      n344 = Get Date/Time In Seconds() -> (seconds since 1Jan1904=w393:timestamp)
                      n345 = Increment(x=w389) -> (x+1=w388:i32)
                      n346 = Format Date/Time String(time format string (%c)="%Y%m%d%H%M%S%3u" ("时间格式字符串(%c)"), seconds (now)=w393) -> (date/time string=w392:string)  [unwired: 1 in]
                      n347 = global write "全局 小时数据发送次数.vi" "小时数据发送次数"(w388) -> ()
                      n348 = Search and Replace String(input string=w392, search string="." ("搜索字符串")) -> (result string=w390:string)  [unwired: 6 in, 3 out]
                      n349 = global read "断电保存全局.vi" "MN"() -> (w384:string)
                      n350 = global read "断电保存全局.vi" "PW"() -> (w383:string)
                      n351 = global read "全局 数据数组大小.vi" "数据数组大小"() -> (w379:i32)
                      n352 = call "数据编码.vi"("table输入"="仪器参数" ("新元素/子数组"), "QN"=w390, "MN"=w384, "PW"=w383) -> ("错误常量"=w382:errorcluster, "通讯包字符串"=w387:string)  [unwired: 10 in]
                      n353 = global read "全局 小时数据发送次数.vi" "小时数据发送次数"() -> (w380:i32)
                      n354 = global write "全局1.vi" "发送报文显示"(w387) -> ()
                      n355 = call "通信状态入队列.vi"("错误输入（无错误）"=w382, "枚举"=enum16{"打开连接", "发送数据", "读取数据", "数据处理", "关闭连接"}."发送数据") -> ()  [unwired: 9 in, 1 out]
                      n356 = Decrement(x=w379) -> (x-1=w378:i32)
                      n357 = Greater Or Equal?(x=w380, y=w378) -> (x >= y?=w377:bool)
                      n358 = Wait (ms)(milliseconds to wait=u32 500 ("等待时间（毫秒）")) -> ()  [unwired: 1 out]
                    }
                  }
                }
              }
              frame True {
              }
            }
          }
        }
      }
      frame "系统状态" {
        # "直接1分钟查询 一次,有变化就按上传,没变化就不上传"
        n359 = flat-sequence {
          frame #0 {
            # "时间"
            n360 = global write "全局 小时数据发送次数.vi" "小时数据发送次数"(0 ("小时数据发送次数")) -> ()
            n361 = global write "全局 数据数组大小.vi" "数据数组大小"(1 ("数据数组大小")) -> ()
            n362 = global write "全局1.vi" "枚举"(enum16{"返回请求应答", "上传数据", "返回执行结果"}."上传数据" ("枚举")) -> ()
          }
          frame #1 {
            # "判定是否存表"
            n363 = global read "全局 数据发送重叠.vi" "掉线指示灯"() -> (w400:bool)
            n364 = case shown="假" w400 {
              frame False {
                n365 = global read "全局1.vi" "系统状态"() -> (w401:bool)
                n366 = case shown="真" w401 {
                  frame False {
                  }
                  frame True {
                    n367 = global read "全局 小时数据发送次数.vi" "小时数据发送次数"() -> (w410:i32)
                    n368 = local write "核查数据上传"(TRUE ("数据上传")) -> ()
                    n369 = global write "全局1.vi" "系统状态"(FALSE ("系统状态")) -> ()
                    n370 = Get Date/Time In Seconds() -> (seconds since 1Jan1904=w414:timestamp)
                    n371 = Increment(x=w410) -> (x+1=w409:i32)
                    n372 = Format Date/Time String(time format string (%c)="%Y%m%d%H%M%S%3u" ("时间格式字符串(%c)"), seconds (now)=w414) -> (date/time string=w413:string)  [unwired: 1 in]
                    n373 = global write "全局 小时数据发送次数.vi" "小时数据发送次数"(w409) -> ()
                    n374 = Search and Replace String(input string=w413, search string="." ("搜索字符串")) -> (result string=w411:string)  [unwired: 6 in, 3 out]
                    n375 = global read "断电保存全局.vi" "MN"() -> (w405:string)
                    n376 = global read "断电保存全局.vi" "PW"() -> (w404:string)
                    n377 = call "数据编码.vi"("table输入"="系统状态" ("新元素/子数组"), "QN"=w411, "MN"=w405, "PW"=w404) -> ("错误常量"=w403:errorcluster, "通讯包字符串"=w408:string)  [unwired: 10 in]
                    n378 = call "通信状态入队列.vi"("错误输入（无错误）"=w403, "枚举"=enum16{"打开连接", "发送数据", "读取数据", "数据处理", "关闭连接"}."发送数据") -> ()  [unwired: 9 in, 1 out]
                    n379 = global write "全局1.vi" "发送报文显示"(w408) -> ()
                  }
                }
              }
              frame True {
              }
            }
          }
        }
      }
      frame "运行模式" {
        # "直接1分钟查询 一次,有变化就按上传,没变化就不上传"
        n380 = flat-sequence {
          frame #0 {
            # "时间"
            n381 = global write "全局 小时数据发送次数.vi" "小时数据发送次数"(0 ("小时数据发送次数")) -> ()
            n382 = global write "全局 数据数组大小.vi" "数据数组大小"(1 ("数据数组大小")) -> ()
            n383 = global write "全局1.vi" "枚举"(enum16{"返回请求应答", "上传数据", "返回执行结果"}."上传数据" ("枚举")) -> ()
          }
          frame #1 {
            # "判定是否存表"
            n384 = global read "全局 数据发送重叠.vi" "掉线指示灯"() -> (w421:bool)
            n385 = case shown="假" w421 {
              frame False {
                n386 = global read "全局1.vi" "运行模式"() -> (w422:bool)
                n387 = case shown="真" w422 {
                  frame False {
                  }
                  frame True {
                    n388 = global read "全局 小时数据发送次数.vi" "小时数据发送次数"() -> (w431:i32)
                    n389 = global write "全局1.vi" "运行模式"(FALSE ("系统状态")) -> ()
                    n390 = local write "核查数据上传"(TRUE ("数据上传")) -> ()
                    n391 = Get Date/Time In Seconds() -> (seconds since 1Jan1904=w435:timestamp)
                    n392 = Increment(x=w431) -> (x+1=w430:i32)
                    n393 = Format Date/Time String(time format string (%c)="%Y%m%d%H%M%S%3u" ("时间格式字符串(%c)"), seconds (now)=w435) -> (date/time string=w434:string)  [unwired: 1 in]
                    n394 = global write "全局 小时数据发送次数.vi" "小时数据发送次数"(w430) -> ()
                    n395 = Search and Replace String(input string=w434, search string="." ("搜索字符串")) -> (result string=w432:string)  [unwired: 6 in, 3 out]
                    n396 = global read "断电保存全局.vi" "MN"() -> (w426:string)
                    n397 = global read "断电保存全局.vi" "PW"() -> (w425:string)
                    n398 = call "数据编码.vi"("table输入"="运行模式" ("新元素/子数组"), "QN"=w432, "MN"=w426, "PW"=w425) -> ("错误常量"=w424:errorcluster, "通讯包字符串"=w429:string)  [unwired: 10 in]
                    n399 = call "通信状态入队列.vi"("错误输入（无错误）"=w424, "枚举"=enum16{"打开连接", "发送数据", "读取数据", "数据处理", "关闭连接"}."发送数据") -> ()  [unwired: 9 in, 1 out]
                    n400 = global write "全局1.vi" "发送报文显示"(w429) -> ()
                  }
                }
              }
              frame True {
              }
            }
          }
        }
      }
      frame "测量周期" {
        # "直接1分钟查询 一次,有变化就按上传,没变化就不上传"
        n401 = flat-sequence {
          frame #0 {
            # "时间"
            n402 = global write "全局 小时数据发送次数.vi" "小时数据发送次数"(0 ("小时数据发送次数")) -> ()
            n403 = global write "全局 数据数组大小.vi" "数据数组大小"(1 ("数据数组大小")) -> ()
            n404 = global write "全局1.vi" "枚举"(enum16{"返回请求应答", "上传数据", "返回执行结果"}."上传数据" ("枚举")) -> ()
          }
          frame #1 {
            # "判定是否存表"
            n405 = global read "全局 数据发送重叠.vi" "掉线指示灯"() -> (w442:bool)
            n406 = case shown="假" w442 {
              frame False {
                n407 = global read "全局1.vi" "测量周期"() -> (w443:bool)
                n408 = case shown="真" w443 {
                  frame False {
                  }
                  frame True {
                    n409 = global read "全局 小时数据发送次数.vi" "小时数据发送次数"() -> (w452:i32)
                    n410 = global write "全局1.vi" "测量周期"(FALSE ("系统状态")) -> ()
                    n411 = local write "核查数据上传"(TRUE ("数据上传")) -> ()
                    n412 = Get Date/Time In Seconds() -> (seconds since 1Jan1904=w456:timestamp)
                    n413 = Increment(x=w452) -> (x+1=w451:i32)
                    n414 = Format Date/Time String(time format string (%c)="%Y%m%d%H%M%S%3u" ("时间格式字符串(%c)"), seconds (now)=w456) -> (date/time string=w455:string)  [unwired: 1 in]
                    n415 = global write "全局 小时数据发送次数.vi" "小时数据发送次数"(w451) -> ()
                    n416 = Search and Replace String(input string=w455, search string="." ("搜索字符串")) -> (result string=w453:string)  [unwired: 6 in, 3 out]
                    n417 = global read "断电保存全局.vi" "MN"() -> (w447:string)
                    n418 = global read "断电保存全局.vi" "PW"() -> (w446:string)
                    n419 = call "数据编码.vi"("table输入"="测量周期" ("新元素/子数组"), "QN"=w453, "MN"=w447, "PW"=w446) -> ("错误常量"=w445:errorcluster, "通讯包字符串"=w450:string)  [unwired: 10 in]
                    n420 = global write "全局1.vi" "发送报文显示"(w450) -> ()
                    n421 = call "通信状态入队列.vi"("错误输入（无错误）"=w445, "枚举"=enum16{"打开连接", "发送数据", "读取数据", "数据处理", "关闭连接"}."发送数据") -> ()  [unwired: 9 in, 1 out]
                  }
                }
              }
              frame True {
              }
            }
          }
        }
      }
      frame "超标留样" {
        # "直接1分钟查询 一次,有变化就按上传,没变化就不上传"
        n422 = flat-sequence {
          frame #0 {
            # "时间"
            n423 = global write "全局 小时数据发送次数.vi" "小时数据发送次数"(0 ("小时数据发送次数")) -> ()
            n424 = global write "全局 数据数组大小.vi" "数据数组大小"(1 ("数据数组大小")) -> ()
            n425 = global write "全局1.vi" "枚举"(enum16{"返回请求应答", "上传数据", "返回执行结果"}."上传数据" ("枚举")) -> ()
          }
          frame #1 {
            # "判定是否存表"
            n426 = global read "全局 数据发送重叠.vi" "掉线指示灯"() -> (w463:bool)
            n427 = case shown="假" w463 {
              frame False {
                n428 = global read "全局1.vi" "超标留样"() -> (w464:bool)
                n429 = case shown="真" w464 {
                  frame False {
                  }
                  frame True {
                    n430 = global read "全局 小时数据发送次数.vi" "小时数据发送次数"() -> (w473:i32)
                    n431 = local write "核查数据上传"(TRUE ("数据上传")) -> ()
                    n432 = global write "全局1.vi" "超标留样"(FALSE ("系统状态")) -> ()
                    n433 = Get Date/Time In Seconds() -> (seconds since 1Jan1904=w477:timestamp)
                    n434 = Increment(x=w473) -> (x+1=w472:i32)
                    n435 = Format Date/Time String(time format string (%c)="%Y%m%d%H%M%S%3u" ("时间格式字符串(%c)"), seconds (now)=w477) -> (date/time string=w476:string)  [unwired: 1 in]
                    n436 = global write "全局 小时数据发送次数.vi" "小时数据发送次数"(w472) -> ()
                    n437 = Search and Replace String(input string=w476, search string="." ("搜索字符串")) -> (result string=w474:string)  [unwired: 6 in, 3 out]
                    n438 = global read "断电保存全局.vi" "MN"() -> (w467:string)
                    n439 = global read "断电保存全局.vi" "PW"() -> (w466:string)
                    n440 = call "数据编码.vi"("table输入"="超标留样" ("新元素/子数组"), "QN"=w474, "MN"=w467, "PW"=w466) -> ("错误常量"=w468:errorcluster, "通讯包字符串"=w471:string)  [unwired: 10 in]
                    n441 = global write "全局1.vi" "发送报文显示"(w471) -> ()
                    n442 = call "通信状态入队列.vi"("错误输入（无错误）"=w468, "枚举"=enum16{"打开连接", "发送数据", "读取数据", "数据处理", "关闭连接"}."发送数据") -> ()  [unwired: 9 in, 1 out]
                  }
                }
              }
              frame True {
              }
            }
          }
        }
      }
      frame "报警信息" {
        # "间隔时间上传"
        # "直接1分钟查询 一次,有数据就按数据上传,没数据为空的不传,在数据发送那边有做处理"
        n443 = flat-sequence {
          frame #0 {
            # "分钟时间间隔"
            n444 = call "日志信息主动发送(子VI).vi"() -> ()  [unwired: 12 in]
            n445 = global write "全局 小时数据发送次数.vi" "小时数据发送次数"(0 ("小时数据发送次数")) -> ()
            n446 = global write "全局1.vi" "枚举"(enum16{"返回请求应答", "上传数据", "返回执行结果"}."上传数据" ("枚举")) -> ()
          }
          frame #1 {
            n447 = call "获取报警信息 (子VI).vi"() -> ()  [unwired: 12 in]
          }
          frame #2 {
            n448 = call "数据处理整合 (子VI).vi"("枚举"=enum16{"实时数据排序", "小时数据排序"}."实时数据排序") -> ("已排序的数组"=w485:string[])  [unwired: 10 in]
            n449 = Array Size(array=w485) -> (size(s)=w484:i32)
            n450 = global write "全局 数据数组大小.vi" "数据数组大小"(w484) -> ()
          }
          frame #3 {
            # "判定是否存表"
            n451 = global read "全局 数据发送重叠.vi" "掉线指示灯"() -> (w486:bool)
            n452 = case shown="假" w486 {
              frame False {
                # "判定数据不为空才发"
                n453 = global read "全局 数据数组大小.vi" "数据数组大小"() -> (w487:i32)
                n454 = Greater Than 0?(x=w487) -> (x > 0?=w488:bool)
                n455 = case shown="真" w488 {
                  frame False {
                    n456 = local write "核查数据上传"(FALSE ("数据上传")) -> ()
                  }
                  frame True {
                    n457 = while {
                      stop <- w491 stop-if-true
                      n458 = global read "全局 小时数据发送次数.vi" "小时数据发送次数"() -> (w501:i32)
                      n459 = Wait (ms)(milliseconds to wait=u32 500 ("等待时间（毫秒）")) -> ()  [unwired: 1 out]
                      n460 = Get Date/Time In Seconds() -> (seconds since 1Jan1904=w505:timestamp)
                      n461 = Increment(x=w501) -> (x+1=w500:i32)
                      n462 = Format Date/Time String(time format string (%c)="%Y%m%d%H%M%S%3u" ("时间格式字符串(%c)"), seconds (now)=w505) -> (date/time string=w504:string)  [unwired: 1 in]
                      n463 = global write "全局 小时数据发送次数.vi" "小时数据发送次数"(w500) -> ()
                      n464 = global read "全局 数据数组大小.vi" "数据数组大小"() -> (w493:i32)
                      n465 = Search and Replace String(input string=w504, search string="." ("搜索字符串")) -> (result string=w502:string)  [unwired: 6 in, 3 out]
                      n466 = global read "断电保存全局.vi" "MN"() -> (w497:string)
                      n467 = global read "断电保存全局.vi" "PW"() -> (w496:string)
                      n468 = global read "全局 小时数据发送次数.vi" "小时数据发送次数"() -> (w494:i32)
                      n469 = call "数据编码.vi"("table输入"="报警信息" ("新元素/子数组"), "QN"=w502, "MN"=w497, "PW"=w496) -> ("错误常量"=w495:errorcluster, "通讯包字符串"=w499:string)  [unwired: 10 in]
                      n470 = Decrement(x=w493) -> (x-1=w492:i32)
                      n471 = global write "全局1.vi" "发送报文显示"(w499) -> ()
                      n472 = Greater Or Equal?(x=w494, y=w492) -> (x >= y?=w491:bool)
                      n473 = call "通信状态入队列.vi"("错误输入（无错误）"=w495, "枚举"=enum16{"打开连接", "发送数据", "读取数据", "数据处理", "关闭连接"}."发送数据") -> ()  [unwired: 9 in, 1 out]
                    }
                  }
                }
              }
              frame True {
              }
            }
          }
        }
      }
      frame "环境参数" {
      }
    }
  }
  "错误输出" <- w1
